vi "Rename Controls.vi"(8 "error in (no error)":errorcluster, 10 "VI Reference":refnum<vi>, 11 "ProjectItem in":refnum<class "ProjectItem.lvclass">) -> (0 "error out":errorcluster, 1 "Changed?":bool, 2 "VI Reference out":refnum<vi>, 3 "ProjectItem out":refnum<class "ProjectItem.lvclass">)   [LabVIEW 2019, in "ProjectItem.lvclass"]
uses:
  ProjectItem.lvclass
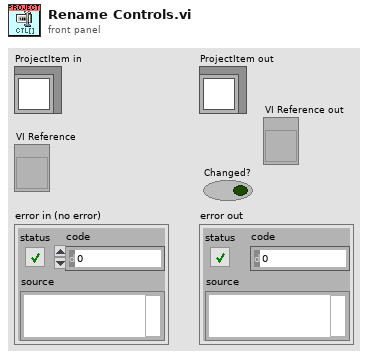
[diagram p1: front panel]
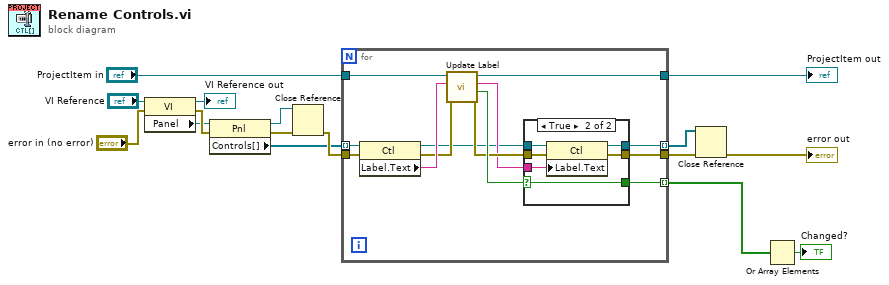
[diagram p0: block diagram]
diagram:
  n1 = property class="VI"(reference="VI Reference", error in="error in (no error)") -> (reference out=→"VI Reference out":refnum<vi>, error out=w15:errorcluster, "Panel"=w7:refnum<vi>)
  n2 = property class="Pnl"(reference=w7, error in=w15) -> (reference out=w9:refnum<vi>, error out=w10:errorcluster, "Controls[]"=w8:refnum<vi>[])
  n3 = Close Reference(reference=w9, error in (no error)=w10) -> (error out=w16:errorcluster)
  n4 = for {
    tunnel: "ProjectItem in" -> [w29]
    tunnel: [w28] -> w5
    tunnel: [w27] -> w3 mode=indexing
    tunnel: [w26] -> w11 mode=indexing
    tunnel: [w25] -> w12
    tunnel: w8 -> [w24] mode=indexing
    tunnel: w16 -> [w17]
    n5 = property class="Ctl"(reference=w24, error in=w17) -> (reference out=w18:refnum<vi>, error out=w19:errorcluster, "Label.Text"=w20:string)
    n6 = call "Update Label.vi"("error in (no error)"=w19, "Label in"=w20, "Rename in"=w29) -> ("error out"=w22:errorcluster, "New Label?"=w23:bool, "Label out"=w21:string, "Rename out"=w28:refnum<class "ProjectItem.lvclass">)  [unwired: 5 in]
    n7 = case shown="True" w23 {
      selector: w23 -> [w32 w35]
      tunnel: w18 -> [w31 w38]
      tunnel: w21 -> [_ w37]
      tunnel: w22 -> [w30 w36]
      tunnel: [w32 w35] -> w27
      tunnel: [w31 w34] -> w26
      tunnel: [w30 w33] -> w25
      frame False {
      }
      frame True {
        n8 = property class="Ctl"(reference=w38, error in=w36, "Label.Text"=w37) -> (reference out=w34:refnum<vi>, error out=w33:errorcluster)
      }
    }
  }
  "ProjectItem out" <- w5
  n9 = Close Reference(reference=w11, error in (no error)=w12) -> (error out=→"error out":errorcluster)
  n10 = Or Array Elements(Boolean array=w3) -> (logical OR=→"Changed?":bool)
